vi "Load Target.vi"(7 "Number of Bits (n)":u32, 8 "error in":errorcluster, 10 "Target String":dbl, 11 "Sentence in":refnum<class "Solution.lvclass">) -> (0 "error out":errorcluster, 3 "Sentence out":refnum<class "Solution.lvclass">)   [LabVIEW 2016, in "Solution.lvclass"]
uses:
  Solution.lvclass
  C:/Users/J51654/My Projects/Evolutionary Programming/GA Framework/IChromosome/IChromosome.lvclass
  Gene/Bit.lvclass
  C:/Users/J51654/My Projects/Evolutionary Programming/GA Framework/IGene/IGene.lvclass
  Gene/Bit.lvclass/Bit.ctl
  IChromosome/IChromosome.lvclass/IChromosome.ctl
  IChromosome/IChromosome.lvclass
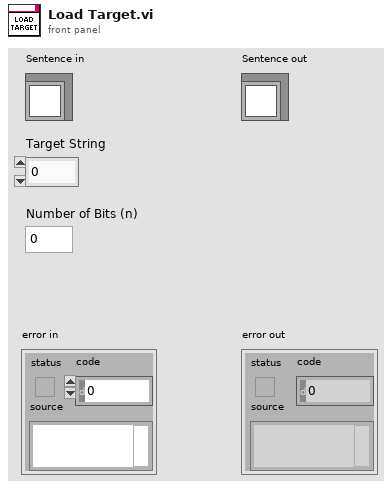
[diagram p1: front panel]
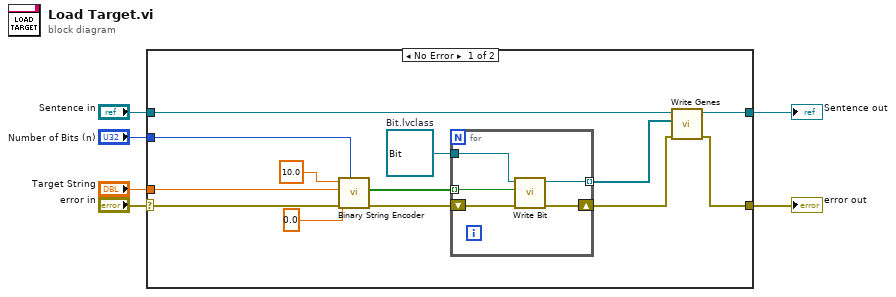
[diagram p0: block diagram]
diagram:
  n1 = case shown="No Error" "error in" {
    selector: "error in" -> [w17 w25]
    tunnel: [w12 w25] -> w5
    tunnel: [w15 w24] -> w3
    tunnel: "Sentence in" -> [w16 w24]
    tunnel: "Target String" -> [w10 _]
    tunnel: "Number of Bits (n)" -> [w7 _]
    frame No Error {
      w18 = refnum<class "Bit.lvclass"> refnum  # Bit.lvclass
      n2 = call "Binary String Encoder.vi"("Number of Bits (n)"=w7, "X_L (0.0)"=0.0, "x"=w10, "X_U (1.0)"=10.0) -> ("Binary String (LSb[0] - MSb[n-1])"=w11:bool[])  [unwired: 7 in]
      n3 = for {
        tunnel: w18 -> [w19]
        tunnel: [w23] -> w14 mode=indexing
        shift-right: [w21] -> w13
        shift-left: w17 -> [w22]
        tunnel: w11 -> [w20] mode=indexing
        n4 = call "Write Bit.vi"("error in (no error)"=w22, "Bit"=w20, "Bit in"=w19) -> ("error out"=w21:errorcluster, "Bit out"=w23:refnum<class "Bit.lvclass">)  [unwired: 7 in]
      }
      n5 = call "Write Genes.vi"("error in"=w13, "Genes"=w14, "IChromosome in"=w16) -> ("error out"=w12:errorcluster, "IChromosome out"=w15:refnum<class "Solution.lvclass">)  [unwired: 7 in]
    }
    frame Error {
    }
  }
  "error out" <- w5
  "Sentence out" <- w3
